vi "time_my.vi"() -> (0 "时间":string)   [LabVIEW 2020]
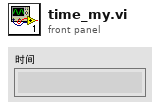
[diagram p1: front panel]
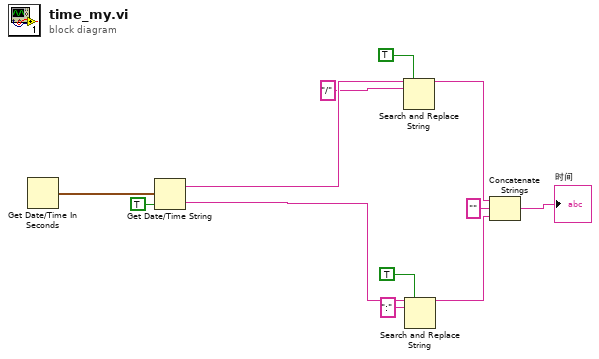
[diagram p0: block diagram]
diagram:
  n1 = Get Date/Time In Seconds() -> (seconds since 1Jan1904=w6:timestamp)
  n2 = Get Date/Time String(seconds (now)=w6, want seconds? (F)=TRUE ("需要秒？(F)")) -> (date string=w12:string, time string=w9:string)  [unwired: 1 in]
  n3 = Search and Replace String(replace all?=TRUE ("替换全部？(F)"), input string=w12, search string="/" ("搜索字符串")) -> (result string=w4:string)  [unwired: 5 in, 3 out]
  n4 = Search and Replace String(replace all?=TRUE ("替换全部？(F)"), input string=w9, search string=":" ("搜索字符串")) -> (result string=w2:string)  [unwired: 5 in, 3 out]
  n5 = Concatenate Strings(w4, "" ("字符串"), w2) -> (→"时间":string)
